vi "Load TDMS Data.vi"(0 "TDMS Path":path, 5 "Cluster":T2, 11 "error in (no error)":errorcluster) -> (4 "G vs Vsg":cluster{"array type (2D Dbl)":dbl[], dbl[]}[](array[cluster]), 6 "Vsg O&M":T1, 8 "B O&M":T1, 10 "B []":dbl[](array[numeric]), 15 "error out":errorcluster)   [LabVIEW 2016, in "Tranconductance SM.lvclass"]
uses:
  Tranconductance SM.lvclass
  <vilib>/Utility/miscctls.llb/LVOffsetAndMultiplierTypeDef.ctl
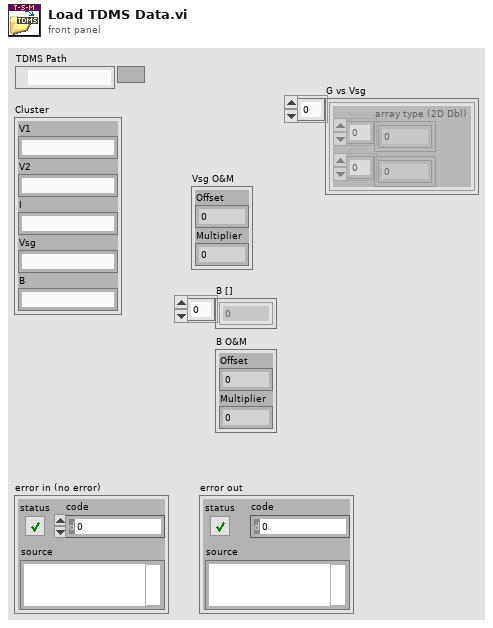
[diagram p1: front panel]
types:
  T1 = typedef "LVOffsetAndMultiplierTypeDef.ctl" = cluster{"Offset":dbl, "Multiplier":dbl}
  T2 = cluster{"V1":string, "V2":string, "I":string, "Vsg":string, "B":string}
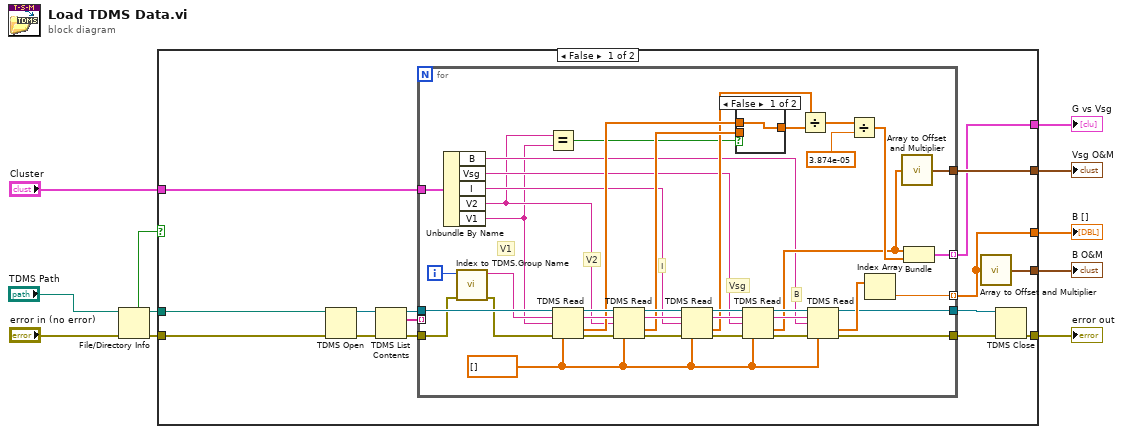
[diagram p0: block diagram]
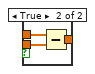
[diagram p2: hidden frame]
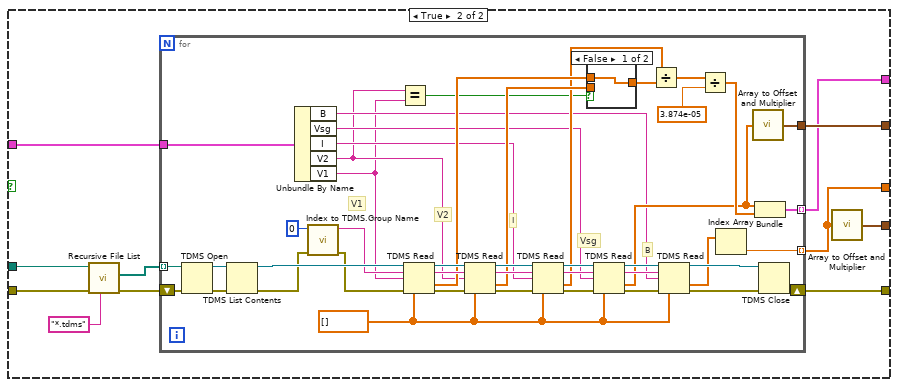
[diagram p3: hidden frame]
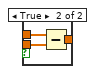
[diagram p4: hidden frame]
diagram:
  n1 = File/Directory Info(path="TDMS Path", error in="error in (no error)") -> (path out=w2:path, directory=w1:bool, error out=w5:errorcluster)  [unwired: 4 out]
  n2 = case shown="False" w1 {
    tunnel: [w26 w80] -> w11
    tunnel: "Cluster" -> [w25 w79]
    tunnel: [w24 w78] -> w9
    tunnel: [w23 w77] -> w8
    tunnel: [w22 w76] -> w7
    tunnel: w5 -> [w14 w73]
    tunnel: [w13 w75] -> w3
    tunnel: w2 -> [w12 w72]
    frame False {
      n3 = TDMS Open(8:w14, 11:w12) -> (0:w15:errorcluster, 3:w16:refnum<k34>)  [unwired: 5 in]
      n4 = TDMS List Contents(4:w15, 7:w16) -> (0:w18:errorcluster, 2:w17:string[], 3:w19:refnum<k34>)  [unwired: 1 in, 1 out]
      n5 = for {
        tunnel: w17 -> [_] mode=indexing
        tunnel: w18 -> [w36]
        tunnel: w19 -> [w62]
        tunnel: [w50] -> w26 mode=indexing
        tunnel: [w47] -> w22 mode=indexing
        tunnel: [w45] -> w20
        tunnel: [w44] -> w21
        tunnel: [w39] -> w23
        tunnel: w25 -> [w33]
        i -> [w38]
        w55 = dbl[] [] ("array type (2D Dbl)")
        # "B"
        # "Vsg"
        # "I"
        # "V2"
        # "V1"
        n6 = Unbundle By Name(w33) -> ("B"=w30:string, "Vsg"=w31:string, "I"=w32:string, "V2"=w29:string, "V1"=w28:string)
        n7 = call "Index to TDMS.Group Name.vi"("error in (no error)"=w36, "Append Index"=w38) -> ("error out"=w35:errorcluster, "group name in (Untitled)"=w37:string)  [unwired: 8 in]
        n8 = Equal?(x=w29, y=w28) -> (x = y?=w27:bool)
        n9 = TDMS Read(0:w62, 5:w37, 7:w28, 11:w35, 12:w55) -> (4:w61:refnum<k34>, 6:w54:string, 10:w42:dbl[], 15:w60:errorcluster)  [unwired: 3 in, 2 out]
        n10 = TDMS Read(0:w61, 5:w54, 7:w29, 11:w60, 12:w55) -> (4:w65:refnum<k34>, 6:w64:string, 10:w41:dbl[], 15:w63:errorcluster)  [unwired: 3 in, 2 out]
        n11 = TDMS Read(0:w65, 5:w64, 7:w32, 11:w63, 12:w55) -> (4:w59:refnum<k34>, 6:w53:string, 10:w34:dbl[], 15:w56:errorcluster)  [unwired: 3 in, 2 out]
        n12 = case shown="False" w27 {
          tunnel: [w66 w69] -> w43
          tunnel: w42 -> [w66 w68]
          tunnel: w41 -> [_ w67]
          frame False {
          }
          frame True {
            n13 = Subtract(x=w68, y=w67) -> (x-y=w69:dbl[])
          }
        }
        n14 = TDMS Read(0:w59, 5:w53, 7:w31, 11:w56, 12:w55) -> (4:w58:refnum<k34>, 6:w52:string, 10:w40:dbl[], 15:w57:errorcluster)  [unwired: 3 in, 2 out]
        n15 = Divide(x=w34, y=w43) -> (x/y=w49:dbl[])
        n16 = TDMS Read(0:w58, 5:w52, 7:w30, 11:w57, 12:w55) -> (4:w44:refnum<k34>, 10:w51:dbl[], 15:w45:errorcluster)  [unwired: 3 in, 3 out]
        n17 = Divide(x=w49, y=3.874e-05) -> (x/y=w46:dbl[])
        n18 = Index Array(array=w51) -> (element=w50:dbl)  [unwired: 1 in]
        n19 = call "Array to Offset and Multiplier.vi"("Array"=w40) -> ("Offset and Multiplier"=w39:T1)
        n20 = Bundle("array type (2D Dbl)"=w40, w46) -> (w47:cluster{"array type (2D Dbl)":dbl[], dbl[]})  [unwired: 1 in]
      }
      n21 = call "Array to Offset and Multiplier.vi"("Array"=w26) -> ("Offset and Multiplier"=w24:T1)
      n22 = TDMS Close(8:w20, 11:w21) -> (0:w13:errorcluster)  [unwired: 1 out]
    }
    frame True {
      n23 = call <vilib>:"Recursive File List.vi"("pattern"="*.tdms", "error in (no error)"=w73, "Folder Path"=w72) -> ("error out"=w70:errorcluster, "All Files in Dir"=w71:path[])  [unwired: 4 in, 3 out]
      n24 = for {
        tunnel: [w124] -> w80 mode=indexing
        tunnel: w79 -> [w123]
        tunnel: [w122] -> w77
        tunnel: [w121] -> w76 mode=indexing
        tunnel: w71 -> [w113] mode=indexing
        shift-right: [w114] -> w75
        shift-left: w70 -> [w112]
        w102 = dbl[] [] ("array type (2D Dbl)")
        # "B"
        # "Vsg"
        # "I"
        # "V2"
        # "V1"
        n25 = TDMS Open(8:w112, 11:w113) -> (0:w115:errorcluster, 3:w116:refnum<k34>)  [unwired: 5 in]
        n26 = TDMS List Contents(4:w115, 7:w116) -> (0:w117:errorcluster, 3:w118:refnum<k34>)  [unwired: 1 in, 2 out]
        n27 = Unbundle By Name(w123) -> ("B"=w85:string, "Vsg"=w86:string, "I"=w87:string, "V2"=w83:string, "V1"=w82:string)
        n28 = call "Index to TDMS.Group Name.vi"("error in (no error)"=w117, "Append Index"=0) -> ("error out"=w89:errorcluster, "group name in (Untitled)"=w90:string)  [unwired: 8 in]
        n29 = Equal?(x=w83, y=w82) -> (x = y?=w81:bool)
        n30 = TDMS Read(0:w118, 5:w90, 7:w82, 11:w89, 12:w102) -> (4:w108:refnum<k34>, 6:w101:string, 10:w93:dbl[], 15:w107:errorcluster)  [unwired: 3 in, 2 out]
        n31 = TDMS Read(0:w108, 5:w101, 7:w83, 11:w107, 12:w102) -> (4:w111:refnum<k34>, 6:w110:string, 10:w92:dbl[], 15:w109:errorcluster)  [unwired: 3 in, 2 out]
        n32 = TDMS Read(0:w111, 5:w110, 7:w87, 11:w109, 12:w102) -> (4:w106:refnum<k34>, 6:w100:string, 10:w88:dbl[], 15:w103:errorcluster)  [unwired: 3 in, 2 out]
        n33 = case shown="False" w81 {
          tunnel: [w125 w128] -> w94
          tunnel: w93 -> [w125 w127]
          tunnel: w92 -> [_ w126]
          frame False {
          }
          frame True {
            n34 = Subtract(x=w127, y=w126) -> (x-y=w128:dbl[])
          }
        }
        n35 = TDMS Read(0:w106, 5:w100, 7:w86, 11:w103, 12:w102) -> (4:w105:refnum<k34>, 6:w99:string, 10:w91:dbl[], 15:w104:errorcluster)  [unwired: 3 in, 2 out]
        n36 = Divide(x=w88, y=w94) -> (x/y=w97:dbl[])
        n37 = TDMS Read(0:w105, 5:w99, 7:w85, 11:w104, 12:w102) -> (4:w120:refnum<k34>, 10:w98:dbl[], 15:w119:errorcluster)  [unwired: 3 in, 3 out]
        n38 = Divide(x=w97, y=3.874e-05) -> (x/y=w95:dbl[])
        n39 = Index Array(array=w98) -> (element=w124:dbl)  [unwired: 1 in]
        n40 = call "Array to Offset and Multiplier.vi"("Array"=w91) -> ("Offset and Multiplier"=w122:T1)
        n41 = Bundle("array type (2D Dbl)"=w91, w95) -> (w121:cluster{"array type (2D Dbl)":dbl[], dbl[]})  [unwired: 1 in]
        n42 = TDMS Close(8:w119, 11:w120) -> (0:w114:errorcluster)  [unwired: 1 out]
      }
      n43 = call "Array to Offset and Multiplier.vi"("Array"=w80) -> ("Offset and Multiplier"=w78:T1)
    }
  }
  "B []" <- w11
  "B O&M" <- w9
  "Vsg O&M" <- w8
  "G vs Vsg" <- w7
  "error out" <- w3
